vi "CRYWork Before Step Close.vi"(11 "StepVI Ref":refnum<vi>) -> ()   [LabVIEW 2013]
uses:
  CRYStepSetup/CRYStepSetup Global.vi
  CRYWindow/SubVI/CRYMain Sub Window Global.vi
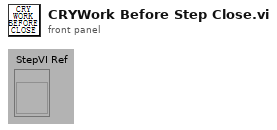
[diagram p1: front panel]
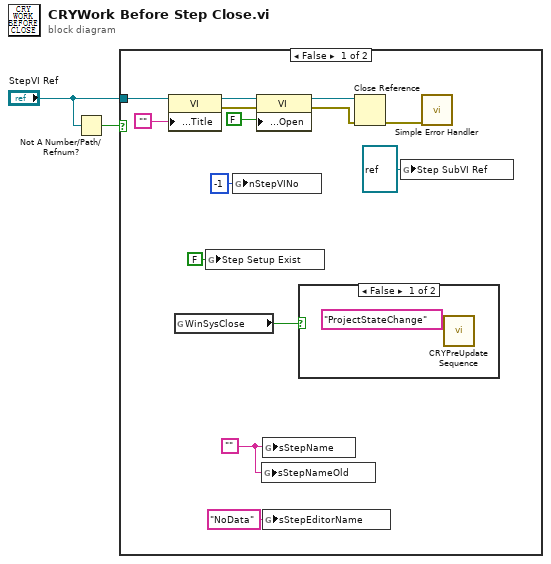
[diagram p0: block diagram]
diagram:
  n1 = Not A Number/Path/Refnum?(number/path/refnum="StepVI Ref") -> (NaN/Path/Refnum?=w1:bool)
  n2 = case shown="False" w1 {
    tunnel: "StepVI Ref" -> [w7 _]
    frame False {
      w3 = ""
      n3 = property class="VI"(reference=w7, "Front Panel.Title"="") -> (reference out=w6:refnum<vi>, error out=w4:errorcluster)  [unwired: 1 in]
      n4 = global read "CRYMain Sub Window Global.vi" "WinSysClose"() -> (w10:bool)
      n5 = global write "CRYStepSetup Global.vi" "Step Setup Exist"(FALSE ("Step Setup Exist")) -> ()
      n6 = global write "CRYStepSetup Global.vi" "nStepVINo"(-1 ("nStepVINo")) -> ()
      n7 = property class="VI"(reference=w6, error in=w4, "Front Panel Window:Open"=FALSE ("Front Panel.Open")) -> (reference out=w15:refnum<vi>, error out=w14:errorcluster)
      n8 = global write "CRYStepSetup Global.vi" "sStepNameOld"(w3) -> ()
      n9 = global write "CRYStepSetup Global.vi" "sStepName"(w3) -> ()
      n10 = global write "CRYStepSetup Global.vi" "sStepEditorName"("NoData" ("sStepEditorName")) -> ()
      n11 = case shown="False" w10 {
        frame False {
          n12 = call "CRYPreUpdate Sequence.vi"("EventName"="ProjectStateChange") -> ()  [unwired: 15 in]
        }
        frame True {
        }
      }
      n13 = Close Reference(reference=w15, error in (no error)=w14) -> (error out=w13:errorcluster)
      n14 = global write "CRYStepSetup Global.vi" "Step SubVI Ref"(refnum<vi> refnum ("Step SubVI Ref")) -> ()
      n15 = call <vilib>:"Simple Error Handler.vi"("error in (no error)"=w13) -> ()  [unwired: 2 in, 7 out]
    }
    frame True {
    }
  }
